vi "Instrument_Setting.vi"(8 "错误输入（无错误）":errorcluster, 9 "id":string[](array[string]), 10 "Get_USB_Resouce":string[](array[string]), 11 "Address Cluster":T1={"SPU"=refnum, "MPM"=[], "Port_Count"=0.0, "MPM_Count"=0.0, "SPU_Resource"=[], "USB_Resource"=[], "MPM_Communicater"="", "MPM_Count"=0.0, "MPM_Address"=[], "MPM_Portnumber"=[], "SPU_DeviveID"="", "MPM_communcation_method"=[], "TSL_sweepstartwave"=0.0, "TSL_sweepstopwave"=0.0, "TSL_Address"="", "TSL_Communicater"="", "TSL"=refnum, "tsl_communcation_method"=3, "TSL_Portnumber"=0.0} {"tsl_communcation_method" items=["GPIB", "C232C", "TCPIP", "USB"]; "MPM_communcation_method" items=["GPIB", "C232C", "TCPIP", "USB"]}) -> (0 "错误输出":errorcluster, 3 "Address Cluster out":T1={"SPU"=refnum, "MPM"=[], "Port_Count"=0.0, "MPM_Count"=0.0, "SPU_Resource"=[], "USB_Resource"=[], "MPM_Communicater"="", "MPM_Count"=0.0, "MPM_Address"=[], "MPM_Portnumber"=[], "SPU_DeviveID"="", "MPM_communcation_method"=[], "TSL_sweepstartwave"=0.0, "TSL_sweepstopwave"=0.0, "TSL_Address"="", "TSL_Communicater"="", "TSL"=refnum, "tsl_communcation_method"=3, "TSL_Portnumber"=0.0} {"tsl_communcation_method" items=["GPIB", "C232C", "TCPIP", "USB"]; "MPM_communcation_method" items=["GPIB", "C232C", "TCPIP", "USB"]})   [LabVIEW 2017]
doc: "Setting Form"
uses:
  CTL/Address Cluster.ctl
  D:/test/ILSTS/LV_IL_Sample/DLL/InstrumentDLL.dll
  DLL/InstrumentDLL.dll
panel:
  out "Boolean":bool=TRUE
  in  "Port_Count":i32
  in  "btnconnect":bool
  in  "cmbSPU_dev":u16(ring) caption="Device" items=["Dev8"]
  in  "IP Address_MPM 2":string caption="IP Address"
  in  "LAN Port_MPM 2":dbl caption="LAN Port"
  in  "GPIB Address_MPM 2":i32 caption="GPIB Address"
  in  "chkmulti_dev":bool
  in  "IP Address_MPM":string caption="IP Address"
  in  "LAN Port_MPM":dbl caption="LAN Port"
  in  "GPIB Address_MPM":i32=14 caption="GPIB Address"
  in  "Communication_MPM":enum32{"rdiGPIB_MPM", "rdiLAN_MPM"}(radio) caption="Communication"
  in  "IP Address_TSL1":string caption="IP Address"
  in  "LAN Port_TSL1":i32 caption="LAN Port"
  in  "GPIB Address_TSL1":i32=1 caption="GPIB Address"
  in  "Usb resouce_TSL1":u16(ring) caption="Usb resouce"
  in  "Communication_TSL1":T2(radio) caption="Communication"
  in  "Product_TSL1":enum32{"rdo550_TSL1", "rdo570_TSL1"}(radio) caption="Product"
  # "TSL"
  # "MPM"
  # "Device1"
  # "Device2"
  # "SPU"
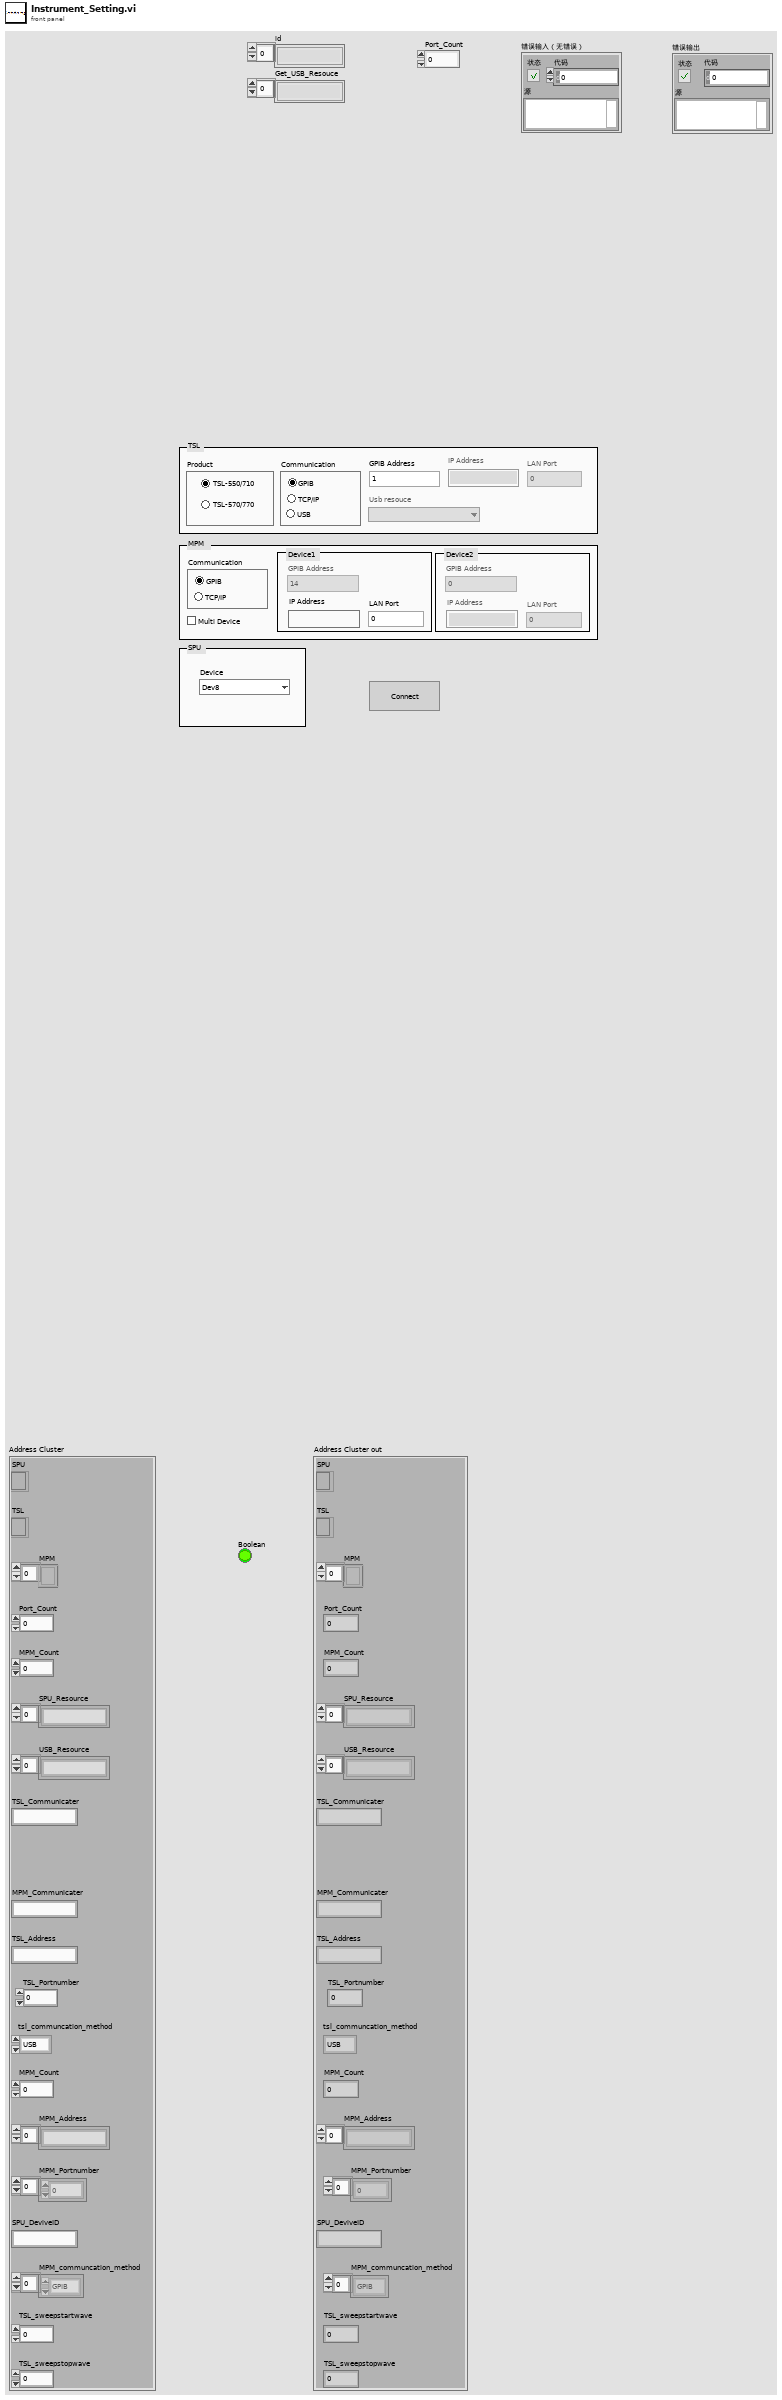
[diagram p1: front panel]
types:
  T1 = typedef "Address Cluster.ctl" = cluster{"SPU":refnum<k24>, "MPM":refnum<k24>[], "Port_Count":dbl, "MPM_Count":dbl, "SPU_Resource":string[], "USB_Resource":string[], "MPM_Communicater":string, "MPM_Count":dbl, "MPM_Address":string[], "MPM_Portnumber":dbl[], "SPU_DeviveID":string, "MPM_communcation_method":i32[], "TSL_sweepstartwave":dbl, "TSL_sweepstopwave":dbl, "TSL_Address":string, "TSL_Communicater":string, "TSL":refnum<k24>, "tsl_communcation_method":i32, "TSL_Portnumber":dbl}
  T2 = enum32{"rdiGPIB_TSL1", "rdiLAN_TSL1", "rdiUSB_TSL1"}
  T3 = enum8{"Enabled", "Disabled", "Disabled and Grayed Out"}
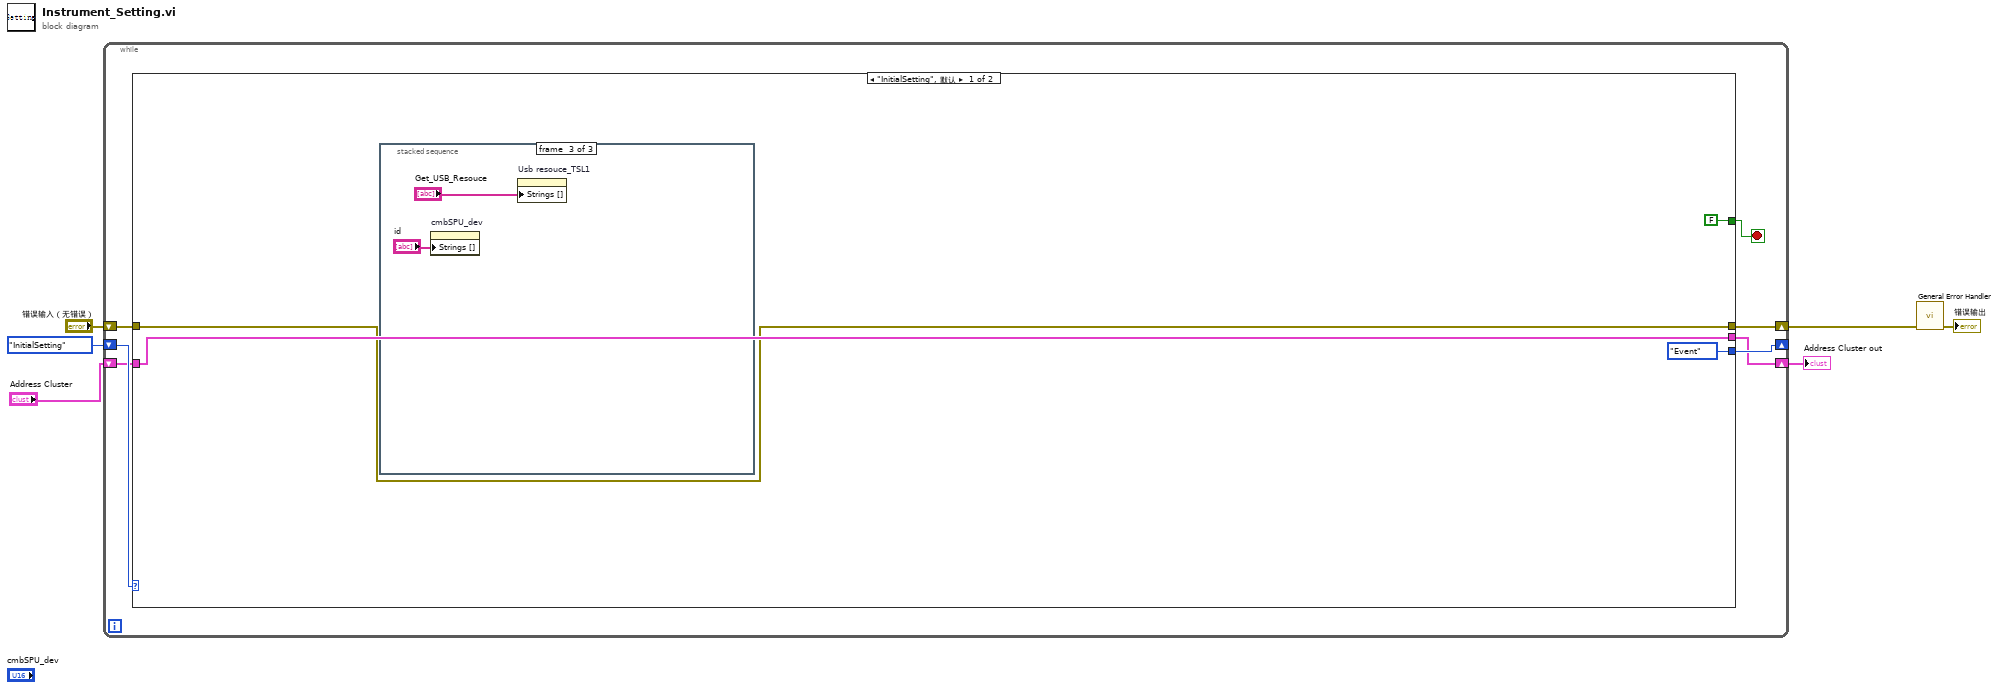
[diagram p0: block diagram]
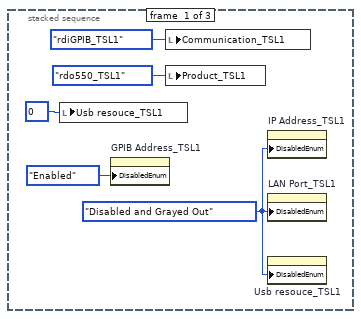
[diagram p2: hidden frame]
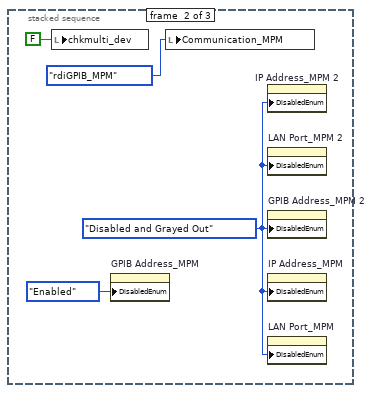
[diagram p3: hidden frame]
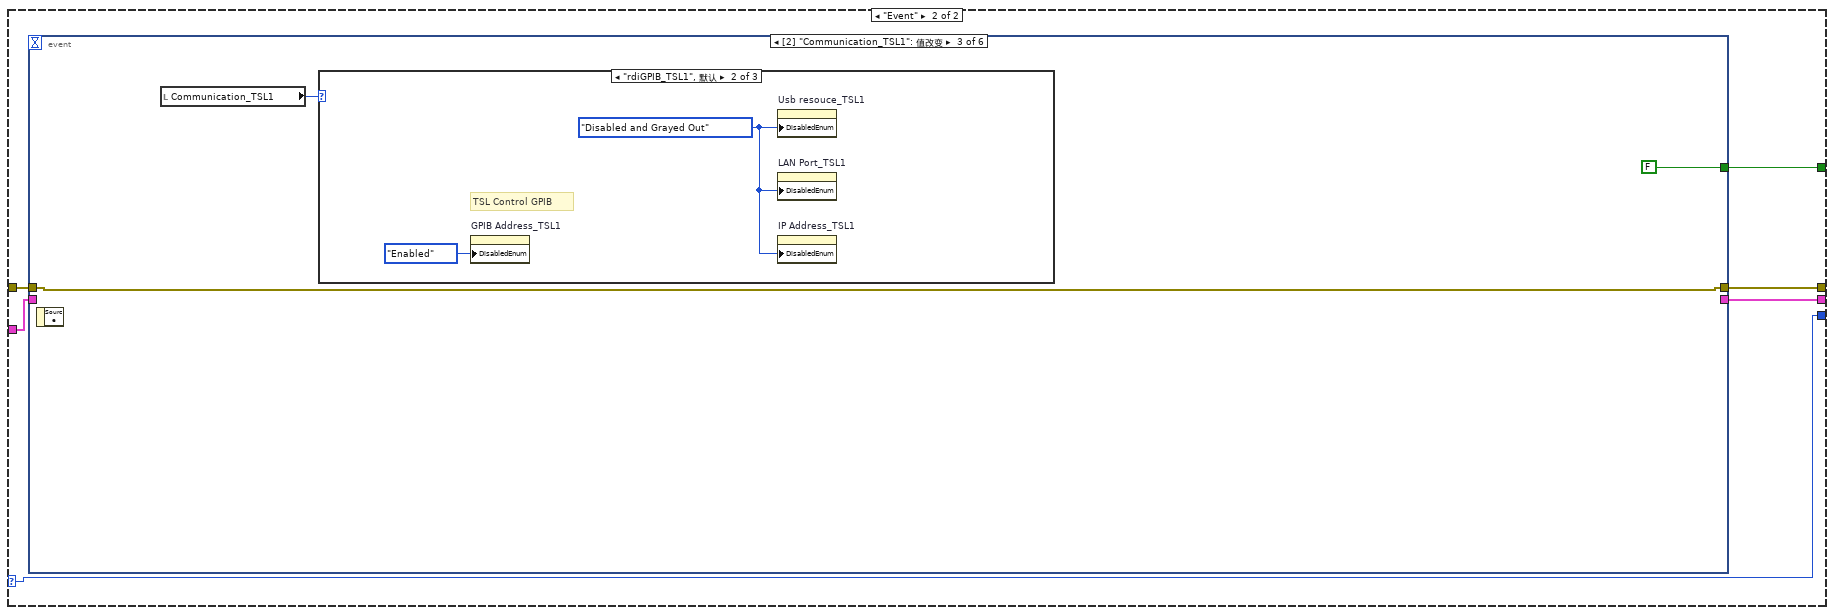
[diagram p4: hidden frame]
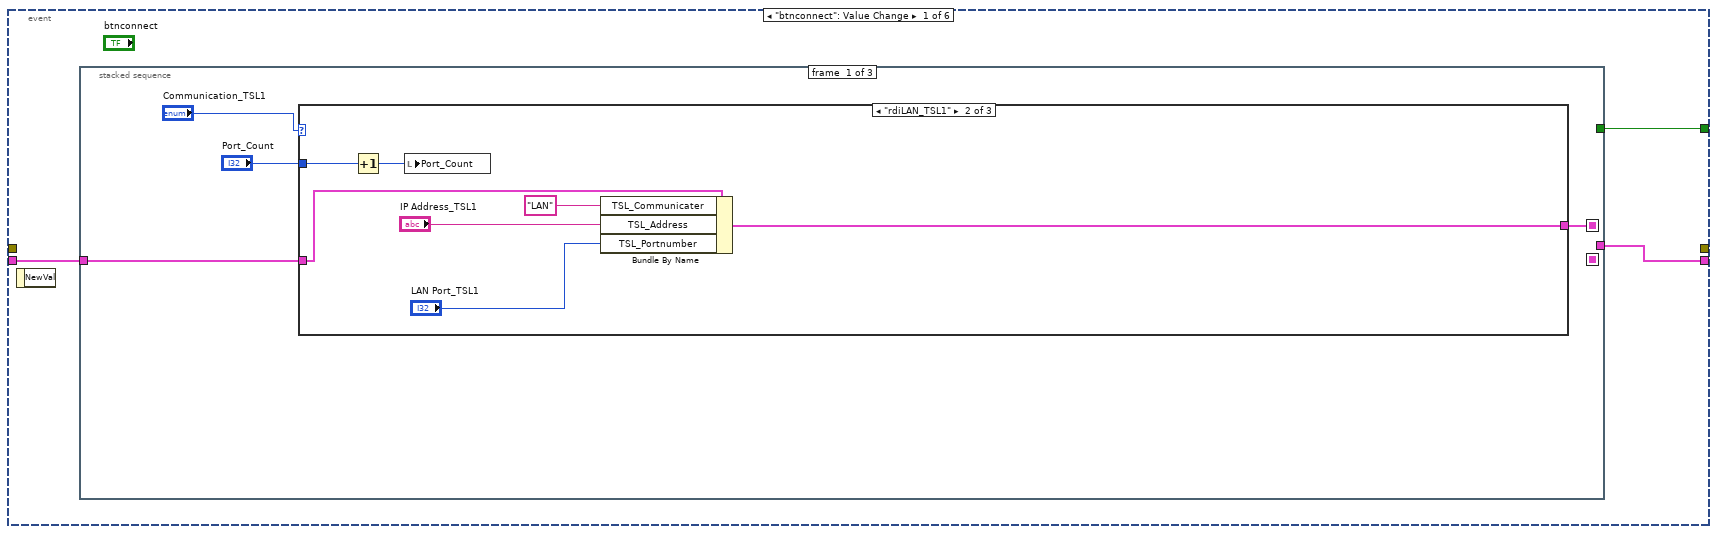
[diagram p5: hidden frame]
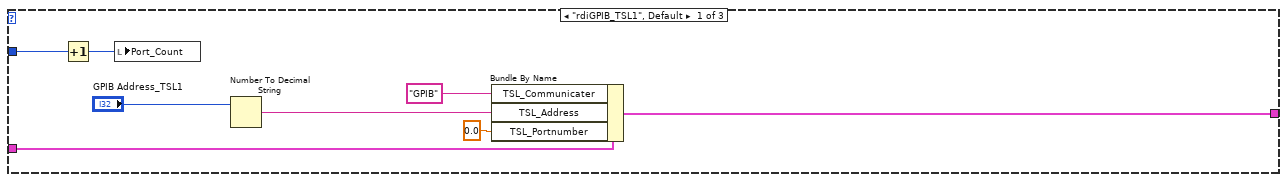
[diagram p6: hidden frame]
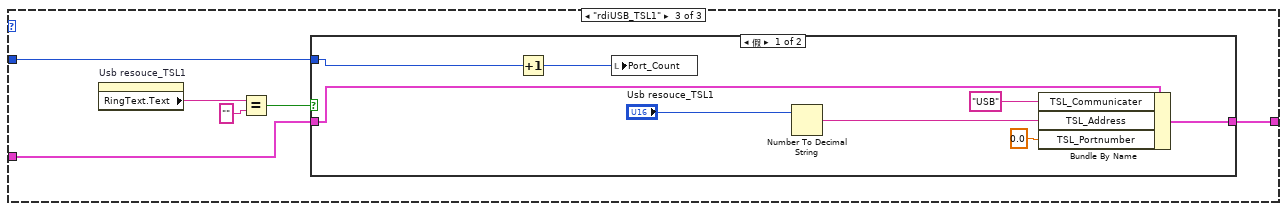
[diagram p7: hidden frame]
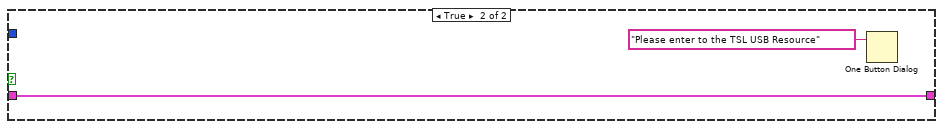
[diagram p8: hidden frame]
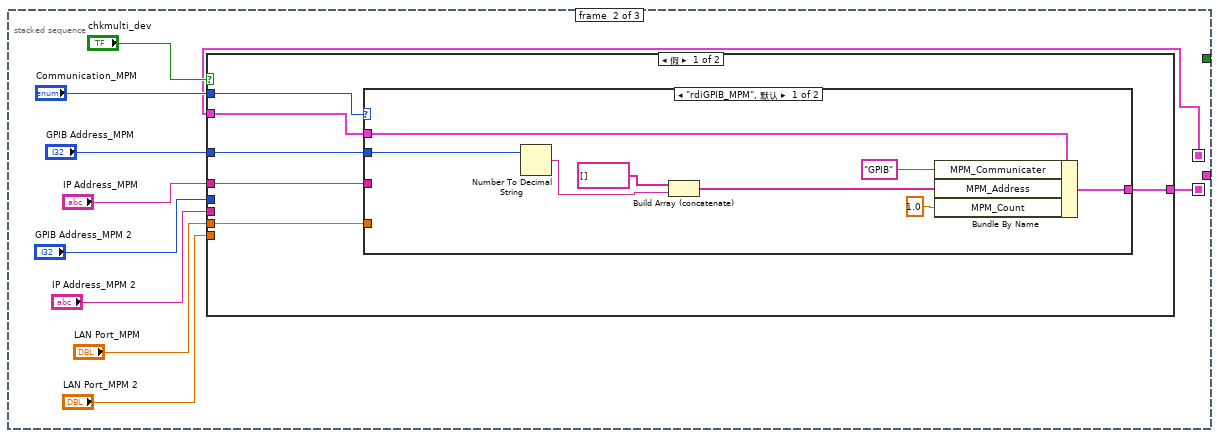
[diagram p9: hidden frame]
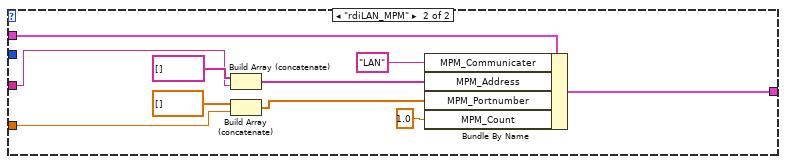
[diagram p10: hidden frame]
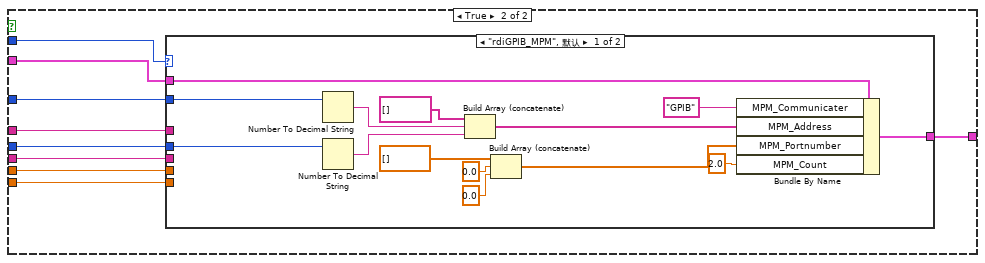
[diagram p11: hidden frame]
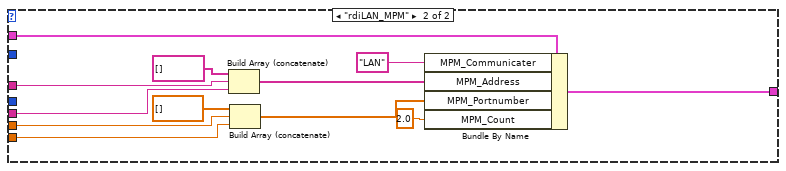
[diagram p12: hidden frame]
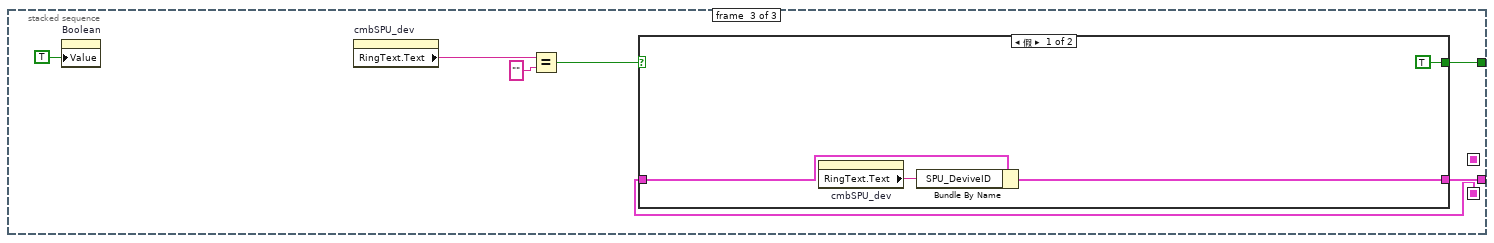
[diagram p13: hidden frame]
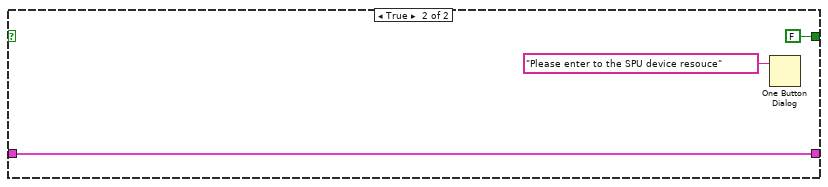
[diagram p14: hidden frame]
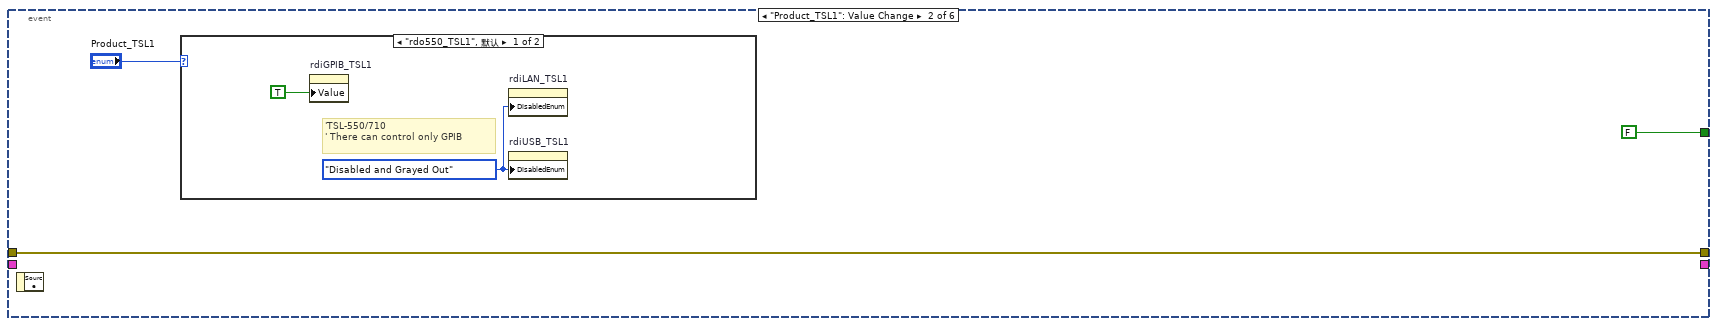
[diagram p15: hidden frame]
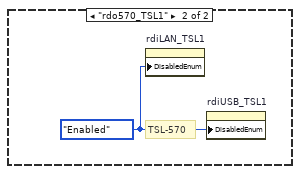
[diagram p16: hidden frame]
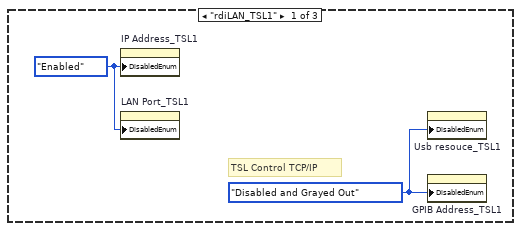
[diagram p17: hidden frame]
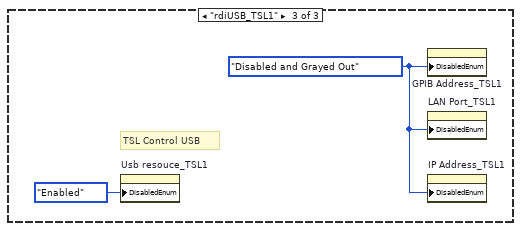
[diagram p18: hidden frame]
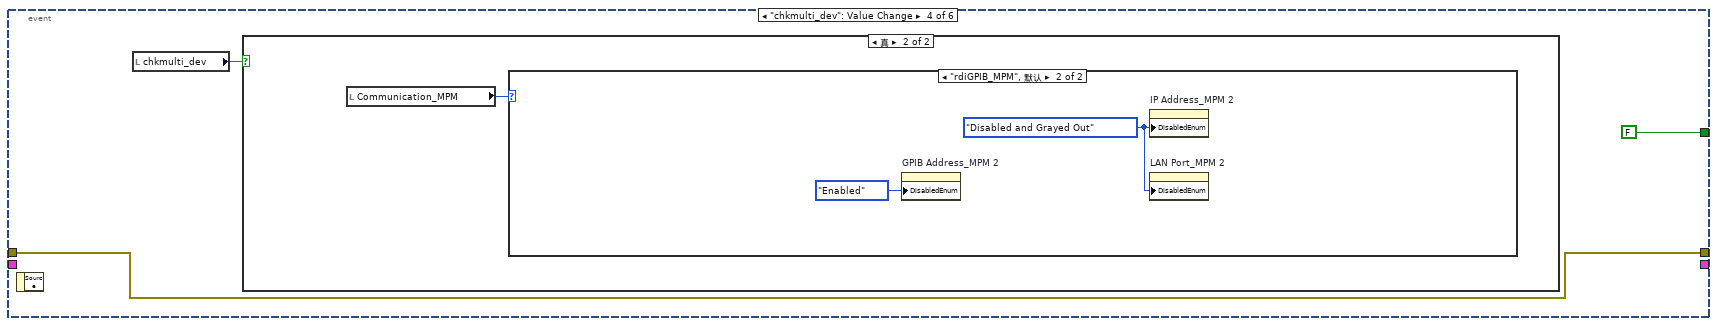
[diagram p19: hidden frame]
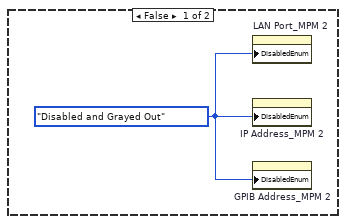
[diagram p20: hidden frame]
diagram:
  n1 = while {
    shift-right: [w12] -> w4
    shift-left: "错误输入（无错误）" -> [w13]
    shift-right: [w10] -> _
    shift-left: enum16{"InitialSetting", "Event", "Set", "Exit"}."InitialSetting" -> [w11]
    shift-right: [w8] -> w1
    shift-left: "Address Cluster" -> [w9]
    stop <- w7 stop-if-true
    n2 = case shown="\"InitialSetting\", 默认" w11 {
      selector: w11 -> [_ w30]
      tunnel: w13 -> [w14 w34]
      tunnel: [w14 w33] -> w12
      tunnel: [FALSE ("status") w29] -> w7
      tunnel: [enum16{"InitialSetting", "Event", "Set", "Exit"}."Event" w30] -> w10
      tunnel: w9 -> [w15 w32]
      tunnel: [w15 w31] -> w8
      frame "InitialSetting", Default {
        n3 = stacked-sequence {
          frame #0 {
            w19 = T3."Disabled and Grayed Out" ("禁用")
            w20 = u16 0 items=[""] ("Usb resouce_TSL1")
            n4 = local write "Usb resouce_TSL1"(w20) -> ()
            n5 = property on="GPIB Address_TSL1" class="DigNum (严格)"("DisabledEnum"=T3."Enabled" ("禁用")) -> ()  [unwired: 2 in, 2 out]
            n6 = local write "Communication_TSL1"(T2."rdiGPIB_TSL1" ("Communication_TSL1")) -> ()
            n7 = local write "Product_TSL1"(enum32{"rdo550_TSL1", "rdo570_TSL1"}."rdo550_TSL1" ("Product_TSL1")) -> ()
            n8 = property on="IP Address_TSL1" class="Str"("DisabledEnum"=w19) -> ()  [unwired: 2 in, 2 out]
            n9 = property on="LAN Port_TSL1" class="DigNum (严格)"("DisabledEnum"=w19) -> ()  [unwired: 2 in, 2 out]
            n10 = property on="Usb resouce_TSL1" class="Ring (严格)"("DisabledEnum"=w19) -> ()  [unwired: 2 in, 2 out]
          }
          frame #1 {
            w23 = T3."Disabled and Grayed Out" ("禁用")
            n11 = local write "chkmulti_dev"(FALSE ("chkmulti_dev")) -> ()
            n12 = property on="GPIB Address_MPM" class="DigNum (严格)"("DisabledEnum"=T3."Enabled" ("禁用")) -> ()  [unwired: 2 in, 2 out]
            n13 = local write "Communication_MPM"(enum32{"rdiGPIB_MPM", "rdiLAN_MPM"}."rdiGPIB_MPM" ("Communication_MPM")) -> ()
            n14 = property on="IP Address_MPM 2" class="Str"("DisabledEnum"=w23) -> ()  [unwired: 2 in, 2 out]
            n15 = property on="LAN Port_MPM 2" class="DigNum (严格)"("DisabledEnum"=w23) -> ()  [unwired: 2 in, 2 out]
            n16 = property on="GPIB Address_MPM 2" class="DigNum (严格)"("DisabledEnum"=w23) -> ()  [unwired: 2 in, 2 out]
            n17 = property on="IP Address_MPM" class="Str"("DisabledEnum"=w23) -> ()  [unwired: 2 in, 2 out]
            n18 = property on="LAN Port_MPM" class="DigNum (严格)"("DisabledEnum"=w23) -> ()  [unwired: 2 in, 2 out]
          }
          frame #2 {
            n19 = property on="cmbSPU_dev" class="Ring (严格)"("Strings []"="id") -> ()  [unwired: 2 in, 2 out]
            n20 = property on="Usb resouce_TSL1" class="Ring (严格)"("Strings []"="Get_USB_Resouce") -> ()  [unwired: 2 in, 2 out]
          }
        }
      }
      frame "Event" {
        n21 = event shown="[2] \"Communication_TSL1\": 值改变" {
          selector: _ -> [_ _ _ _ _ _]
          dyn-events: _ -> [_ _ _ _ _ _]
          timeout: _ -> [_ _ _ _ _ _]
          tunnel: w34 -> [_ w156 w162 w171 w180 _]
          tunnel: [_ w156 w162 w171 w180 _] -> w33
          tunnel: w32 -> [w37 _ _ _ _ w195]
          tunnel: [w36 _ _ _ _ w195] -> w31
          tunnel: [w35 FALSE ("y") FALSE ("y") FALSE ("y") FALSE ("y") TRUE ("y")] -> w29
          event "btnconnect": Value Change {
            n22 = event-data() -> ()  [unwired: 1 in, 1 out]
            n23 = stacked-sequence {
              seq-local: [w40 _ _] -> [_ w73 _]
              seq-local: [_ w74 _] -> [_ _ w143]
              tunnel: w37 -> [w41 _ _]
              tunnel: [_ _ w145] -> w36
              tunnel: [_ _ w144] -> w35
              frame #0 {
                n24 = case shown="\"rdiLAN_TSL1\"" "Communication_TSL1" {
                  tunnel: "Port_Count" -> [w45 w54 w59]
                  tunnel: w41 -> [w48 w56 w58]
                  tunnel: [w47 w55 w57] -> w40
                  frame "rdiGPIB_TSL1", Default {
                    n25 = Increment(x=w45) -> (x+1=w46:i32)
                    n26 = local write "Port_Count"(w46) -> ()
                    n27 = Number To Decimal String(number="GPIB Address_TSL1") -> (decimal integer string=w43:string)  [unwired: 1 in]
                    n28 = Bundle By Name(cluster=w48, "TSL_Communicater"="GPIB" ("新元素/子数组"), "TSL_Address"=w43, "TSL_Portnumber"=0.0 ("新元素/子数组")) -> (w47:T1)
                  }
                  frame "rdiLAN_TSL1" {
                    n29 = Increment(x=w54) -> (x+1=w53:i32)
                    n30 = local write "Port_Count"(w53) -> ()
                    n31 = Bundle By Name(cluster=w56, "TSL_Communicater"="LAN" ("新元素/子数组"), "TSL_Address"="IP Address_TSL1", "TSL_Portnumber"="LAN Port_TSL1") -> (w55:T1)
                  }
                  frame "rdiUSB_TSL1" {
                    n32 = property on="Usb resouce_TSL1" class="Ring (严格)"() -> ("RingText.Text"=w62:string)  [unwired: 2 in, 2 out]
                    n33 = Equal?(x=w62, y="") -> (x = y?=w60:bool)
                    n34 = case shown="假" w60 {
                      tunnel: w59 -> [w66 _]
                      tunnel: w58 -> [w69 w71]
                      tunnel: [w68 w71] -> w57
                      frame False {
                        n35 = Increment(x=w66) -> (x+1=w67:i32)
                        n36 = local write "Port_Count"(w67) -> ()
                        n37 = Number To Decimal String(number="Usb resouce_TSL1") -> (decimal integer string=w64:string)  [unwired: 1 in]
                        n38 = Bundle By Name(cluster=w69, "TSL_Communicater"="USB" ("新元素/子数组"), "TSL_Address"=w64, "TSL_Portnumber"=0.0 ("新元素/子数组")) -> (w68:T1)
                      }
                      frame True {
                        n39 = One Button Dialog(message="Please enter to the TSL USB Resource" ("消息")) -> ()  [unwired: 1 in, 1 out]
                      }
                    }
                  }
                }
              }
              frame #1 {
                n40 = case shown="假" "chkmulti_dev" {
                  tunnel: w73 -> [w84 w115]
                  tunnel: "Communication_MPM" -> [w88 w114]
                  tunnel: [w85 w113] -> w74
                  tunnel: "GPIB Address_MPM 2" -> [_ w112]
                  tunnel: "GPIB Address_MPM" -> [w83 w111]
                  tunnel: "LAN Port_MPM 2" -> [_ w110]
                  tunnel: "LAN Port_MPM" -> [w87 w109]
                  tunnel: "IP Address_MPM 2" -> [_ w108]
                  tunnel: "IP Address_MPM" -> [w86 w107]
                  frame False {
                    n41 = case shown="\"rdiGPIB_MPM\", 默认" w88 {
                      tunnel: w87 -> [_ w103]
                      tunnel: w86 -> [_ w100]
                      tunnel: [w93 w98] -> w85
                      tunnel: w84 -> [w94 w97]
                      tunnel: w83 -> [w90 _]
                      frame "rdiGPIB_MPM", Default {
                        n42 = Number To Decimal String(number=w90) -> (decimal integer string=w91:string)  [unwired: 1 in]
                        n43 = Build Array (concatenate)(string[] [] ("MPM_Address"), w91) -> (w89:string[])
                        n44 = Bundle By Name(cluster=w94, "MPM_Communicater"="GPIB", "MPM_Address"=w89, "MPM_Count"=1.0) -> (w93:T1)
                      }
                      frame "rdiLAN_MPM" {
                        n45 = Build Array (concatenate)(string[] [] ("MPM_Address"), w100) -> (w99:string[])
                        n46 = Build Array (concatenate)(dbl[] [] ("MPM_Portnumber"), w103) -> (w102:dbl[])
                        n47 = Bundle By Name(cluster=w97, "MPM_Communicater"="LAN", "MPM_Address"=w99, "MPM_Portnumber"=w102, "MPM_Count"=1.0) -> (w98:T1)
                      }
                    }
                  }
                  frame True {
                    n48 = case shown="\"rdiGPIB_MPM\", 默认" w114 {
                      tunnel: w115 -> [w123 w141]
                      tunnel: [w118 w130] -> w113
                      tunnel: w112 -> [w117 _]
                      tunnel: w111 -> [w116 _]
                      tunnel: w110 -> [_ w134]
                      tunnel: w109 -> [_ w133]
                      tunnel: w108 -> [_ w132]
                      tunnel: w107 -> [_ w131]
                      frame "rdiGPIB_MPM", Default {
                        n49 = Number To Decimal String(number=w116) -> (decimal integer string=w126:string)  [unwired: 1 in]
                        n50 = Number To Decimal String(number=w117) -> (decimal integer string=w125:string)  [unwired: 1 in]
                        n51 = Build Array (concatenate)(string[] [] ("MPM_Address"), w126, w125) -> (w124:string[])
                        n52 = Build Array (concatenate)(dbl[] [] ("MPM_Portnumber"), 0.0 ("新元素/子数组"), 0.0 ("新元素/子数组")) -> (w119:dbl[])
                        n53 = Bundle By Name(cluster=w123, "MPM_Communicater"="GPIB", "MPM_Address"=w124, "MPM_Portnumber"=w119, "MPM_Count"=2.0) -> (w118:T1)
                      }
                      frame "rdiLAN_MPM" {
                        n54 = Build Array (concatenate)(string[] [] ("MPM_Address"), w131, w132) -> (w137:string[])
                        n55 = Build Array (concatenate)(dbl[] [] ("MPM_Portnumber"), w133, w134) -> (w135:dbl[])
                        n56 = Bundle By Name(cluster=w141, "MPM_Communicater"="LAN", "MPM_Address"=w137, "MPM_Portnumber"=w135, "MPM_Count"=2.0) -> (w130:T1)
                      }
                    }
                  }
                }
              }
              frame #2 {
                n57 = property on="Boolean" class="Bool (严格)"("Value"=TRUE ("Boolean")) -> ()  [unwired: 2 in, 2 out]
                n58 = property on="cmbSPU_dev" class="Ring (严格)"() -> ("RingText.Text"=w147:string)  [unwired: 2 in, 2 out]
                n59 = Equal?(x=w147, y="") -> (x = y?=w148:bool)
                n60 = case shown="假" w148 {
                  tunnel: w143 -> [w152 w154]
                  tunnel: [w151 w154] -> w145
                  tunnel: [TRUE ("y") FALSE ("y")] -> w144
                  frame False {
                    n61 = property on="cmbSPU_dev" class="Ring (严格)"() -> ("RingText.Text"=w150:string)  [unwired: 2 in, 2 out]
                    n62 = Bundle By Name(cluster=w152, "SPU_DeviveID"=w150) -> (w151:T1)
                  }
                  frame True {
                    n63 = One Button Dialog(message="Please enter to the SPU device resouce" ("消息")) -> ()  [unwired: 1 in, 1 out]
                  }
                }
              }
            }
          }
          event "Product_TSL1": Value Change {
            n64 = event-data() -> ()  [unwired: 1 in, 1 out]
            n65 = case shown="\"rdo550_TSL1\", 默认" "Product_TSL1" {
              frame "rdo550_TSL1", Default {
                w160 = T3."Disabled and Grayed Out" ("禁用")
                # "'TSL-550/710\n' There can control only GPIB"
                n66 = property on="rdiGPIB_TSL1" class="Bool (严格)"("Value"=TRUE ("键选中")) -> ()  [unwired: 2 in, 2 out]
                n67 = property on="rdiLAN_TSL1" class="Bool (严格)"("DisabledEnum"=w160) -> ()  [unwired: 2 in, 2 out]
                n68 = property on="rdiUSB_TSL1" class="Bool (严格)"("DisabledEnum"=w160) -> ()  [unwired: 2 in, 2 out]
              }
              frame "rdo570_TSL1" {
                w161 = T3."Enabled" ("禁用")
                # "TSL-570"
                n69 = property on="rdiLAN_TSL1" class="Bool (严格)"("DisabledEnum"=w161) -> ()  [unwired: 2 in, 2 out]
                n70 = property on="rdiUSB_TSL1" class="Bool (严格)"("DisabledEnum"=w161) -> ()  [unwired: 2 in, 2 out]
              }
            }
          }
          event "Communication_TSL1": Value Change {
            n71 = event-data() -> ()  [unwired: 1 in, 1 out]
            n72 = local read "Communication_TSL1"() -> (w164:T2)
            n73 = case shown="\"rdiGPIB_TSL1\", 默认" w164 {
              frame "rdiLAN_TSL1" {
                w165 = T3."Enabled" ("禁用")
                w166 = T3."Disabled and Grayed Out" ("禁用")
                # "TSL Control TCP/IP"
                n74 = property on="IP Address_TSL1" class="Str"("DisabledEnum"=w165) -> ()  [unwired: 2 in, 2 out]
                n75 = property on="LAN Port_TSL1" class="DigNum (严格)"("DisabledEnum"=w165) -> ()  [unwired: 2 in, 2 out]
                n76 = property on="Usb resouce_TSL1" class="Ring (严格)"("DisabledEnum"=w166) -> ()  [unwired: 2 in, 2 out]
                n77 = property on="GPIB Address_TSL1" class="DigNum (严格)"("DisabledEnum"=w166) -> ()  [unwired: 2 in, 2 out]
              }
              frame "rdiGPIB_TSL1", Default {
                w167 = T3."Disabled and Grayed Out" ("禁用")
                # "TSL Control GPIB"
                n78 = property on="GPIB Address_TSL1" class="DigNum (严格)"("DisabledEnum"=T3."Enabled" ("禁用")) -> ()  [unwired: 2 in, 2 out]
                n79 = property on="Usb resouce_TSL1" class="Ring (严格)"("DisabledEnum"=w167) -> ()  [unwired: 2 in, 2 out]
                n80 = property on="LAN Port_TSL1" class="DigNum (严格)"("DisabledEnum"=w167) -> ()  [unwired: 2 in, 2 out]
                n81 = property on="IP Address_TSL1" class="Str"("DisabledEnum"=w167) -> ()  [unwired: 2 in, 2 out]
              }
              frame "rdiUSB_TSL1" {
                w169 = T3."Disabled and Grayed Out" ("禁用")
                # "TSL Control USB"
                n82 = property on="Usb resouce_TSL1" class="Ring (严格)"("DisabledEnum"=T3."Enabled" ("禁用")) -> ()  [unwired: 2 in, 2 out]
                n83 = property on="GPIB Address_TSL1" class="DigNum (严格)"("DisabledEnum"=w169) -> ()  [unwired: 2 in, 2 out]
                n84 = property on="LAN Port_TSL1" class="DigNum (严格)"("DisabledEnum"=w169) -> ()  [unwired: 2 in, 2 out]
                n85 = property on="IP Address_TSL1" class="Str"("DisabledEnum"=w169) -> ()  [unwired: 2 in, 2 out]
              }
            }
          }
          event "chkmulti_dev": Value Change {
            n86 = event-data() -> ()  [unwired: 1 in, 1 out]
            n87 = local read "chkmulti_dev"() -> (w173:bool)
            n88 = case shown="真" w173 {
              frame False {
                w174 = T3."Disabled and Grayed Out" ("禁用")
                n89 = property on="LAN Port_MPM 2" class="DigNum (严格)"("DisabledEnum"=w174) -> ()  [unwired: 2 in, 2 out]
                n90 = property on="IP Address_MPM 2" class="Str"("DisabledEnum"=w174) -> ()  [unwired: 2 in, 2 out]
                n91 = property on="GPIB Address_MPM 2" class="DigNum (严格)"("DisabledEnum"=w174) -> ()  [unwired: 2 in, 2 out]
              }
              frame True {
                n92 = local read "Communication_MPM"() -> (w175:enum32{"rdiGPIB_MPM", "rdiLAN_MPM"})
                n93 = case shown="\"rdiGPIB_MPM\", 默认" w175 {
                  frame "rdiLAN_MPM" {
                    w176 = T3."Enabled" ("禁用")
                    n94 = property on="LAN Port_MPM 2" class="DigNum (严格)"("DisabledEnum"=w176) -> ()  [unwired: 2 in, 2 out]
                    n95 = property on="IP Address_MPM 2" class="Str"("DisabledEnum"=w176) -> ()  [unwired: 2 in, 2 out]
                    n96 = property on="GPIB Address_MPM 2" class="DigNum (严格)"("DisabledEnum"=T3."Disabled and Grayed Out" ("禁用")) -> ()  [unwired: 2 in, 2 out]
                  }
                  frame "rdiGPIB_MPM", Default {
                    w178 = T3."Disabled and Grayed Out" ("禁用")
                    n97 = property on="GPIB Address_MPM 2" class="DigNum (严格)"("DisabledEnum"=T3."Enabled" ("禁用")) -> ()  [unwired: 2 in, 2 out]
                    n98 = property on="IP Address_MPM 2" class="Str"("DisabledEnum"=w178) -> ()  [unwired: 2 in, 2 out]
                    n99 = property on="LAN Port_MPM 2" class="DigNum (严格)"("DisabledEnum"=w178) -> ()  [unwired: 2 in, 2 out]
                  }
                }
              }
            }
          }
          event "Communication_MPM": Value Change {
            n100 = event-data() -> ()  [unwired: 1 in, 1 out]
            n101 = local read "Communication_MPM"() -> (w182:enum32{"rdiGPIB_MPM", "rdiLAN_MPM"})
            n102 = case shown="\"rdiGPIB_MPM\", 默认" w182 {
              frame "rdiLAN_MPM" {
                n103 = local read "chkmulti_dev"() -> (w183:bool)
                n104 = case shown="真" w183 {
                  frame True {
                    w184 = T3."Disabled and Grayed Out" ("禁用")
                    w185 = T3."Enabled" ("禁用")
                    n105 = property on="IP Address_MPM" class="Str"("DisabledEnum"=w185) -> ()  [unwired: 2 in, 2 out]
                    n106 = property on="LAN Port_MPM" class="DigNum (严格)"("DisabledEnum"=w185) -> ()  [unwired: 2 in, 2 out]
                    n107 = property on="LAN Port_MPM 2" class="DigNum (严格)"("DisabledEnum"=w185) -> ()  [unwired: 2 in, 2 out]
                    n108 = property on="IP Address_MPM 2" class="Str"("DisabledEnum"=w185) -> ()  [unwired: 2 in, 2 out]
                    n109 = property on="GPIB Address_MPM 2" class="DigNum (严格)"("DisabledEnum"=w184) -> ()  [unwired: 2 in, 2 out]
                    n110 = property on="GPIB Address_MPM" class="DigNum (严格)"("DisabledEnum"=w184) -> ()  [unwired: 2 in, 2 out]
                  }
                  frame False {
                    w186 = T3."Disabled and Grayed Out" ("禁用")
                    w187 = T3."Disabled and Grayed Out" ("禁用")
                    w188 = T3."Enabled" ("禁用")
                    n111 = property on="IP Address_MPM" class="Str"("DisabledEnum"=w188) -> ()  [unwired: 2 in, 2 out]
                    n112 = property on="LAN Port_MPM" class="DigNum (严格)"("DisabledEnum"=w188) -> ()  [unwired: 2 in, 2 out]
                    n113 = property on="IP Address_MPM 2" class="Str"("DisabledEnum"=w186) -> ()  [unwired: 2 in, 2 out]
                    n114 = property on="LAN Port_MPM 2" class="DigNum (严格)"("DisabledEnum"=w186) -> ()  [unwired: 2 in, 2 out]
                    n115 = property on="GPIB Address_MPM 2" class="DigNum (严格)"("DisabledEnum"=w187) -> ()  [unwired: 2 in, 2 out]
                    n116 = property on="GPIB Address_MPM" class="DigNum (严格)"("DisabledEnum"=w187) -> ()  [unwired: 2 in, 2 out]
                  }
                }
              }
              frame "rdiGPIB_MPM", Default {
                n117 = local read "chkmulti_dev"() -> (w189:bool)
                n118 = case shown="假" w189 {
                  frame True {
                    w190 = T3."Enabled" ("禁用")
                    w191 = T3."Disabled and Grayed Out" ("禁用")
                    n119 = property on="GPIB Address_MPM" class="DigNum (严格)"("DisabledEnum"=w190) -> ()  [unwired: 2 in, 2 out]
                    n120 = property on="GPIB Address_MPM 2" class="DigNum (严格)"("DisabledEnum"=w190) -> ()  [unwired: 2 in, 2 out]
                    n121 = property on="IP Address_MPM" class="Str"("DisabledEnum"=w191) -> ()  [unwired: 2 in, 2 out]
                    n122 = property on="LAN Port_MPM" class="DigNum (严格)"("DisabledEnum"=w191) -> ()  [unwired: 2 in, 2 out]
                    n123 = property on="IP Address_MPM 2" class="Str"("DisabledEnum"=w191) -> ()  [unwired: 2 in, 2 out]
                    n124 = property on="LAN Port_MPM 2" class="DigNum (严格)"("DisabledEnum"=w191) -> ()  [unwired: 2 in, 2 out]
                  }
                  frame False {
                    w192 = T3."Disabled and Grayed Out" ("禁用")
                    n125 = property on="GPIB Address_MPM" class="DigNum (严格)"("DisabledEnum"=T3."Enabled" ("禁用")) -> ()  [unwired: 2 in, 2 out]
                    n126 = property on="GPIB Address_MPM 2" class="DigNum (严格)"("DisabledEnum"=w192) -> ()  [unwired: 2 in, 2 out]
                    n127 = property on="LAN Port_MPM" class="DigNum (严格)"("DisabledEnum"=w192) -> ()  [unwired: 2 in, 2 out]
                    n128 = property on="LAN Port_MPM 2" class="DigNum (严格)"("DisabledEnum"=w192) -> ()  [unwired: 2 in, 2 out]
                    n129 = property on="IP Address_MPM 2" class="Str"("DisabledEnum"=w192) -> ()  [unwired: 2 in, 2 out]
                    n130 = property on="IP Address_MPM" class="Str"("DisabledEnum"=w192) -> ()  [unwired: 2 in, 2 out]
                  }
                }
              }
            }
          }
          event Panel Close? {
            n131 = event-data() -> ()  [unwired: 1 in, 4 out]
            n132 = event-data("Discard?"=TRUE ("放弃？")) -> ()  [unwired: 1 in, 1 out]
            "Boolean" <- FALSE
          }
        }
      }
    }
  }
  "Address Cluster out" <- w1
  n133 = call <vilib>:"General Error Handler.vi"("error in (no error)"=w4) -> ("error out"=→"错误输出":errorcluster)  [unwired: 10 in, 4 out]
